vi "ke37xx Limit Test Results.vi"(0 "VISA Resource Name":refnum<visa-resource-name>, 7 "Clear (False)":bool, 11 "error in (no error)":errorcluster) -> (4 "VISA Resource Name Out":refnum<visa-resource-name>, 6 "Low Limit Failed":bool, 8 "High Limit Failed":bool, 15 "error out":errorcluster)   [LabVIEW 2009, in "Keithley 3700 Series.lvlib"]
doc: "This VI allows you to clear or to query the limit test results."
uses:
  <instrlib>/Keithley 3706/Keithley 3700 Series.lvlib
panel:
  in  "Limit Line (1)":u8=1 min=1 max=2
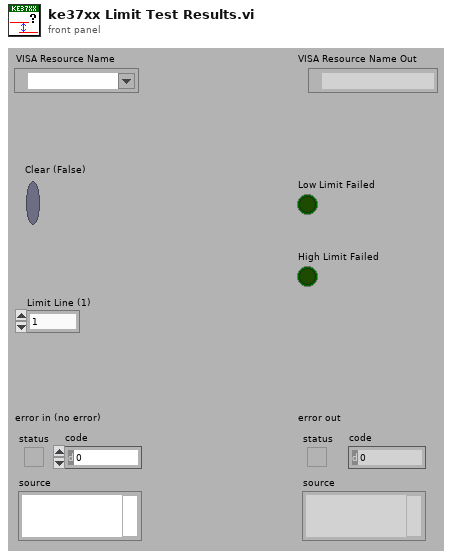
[diagram p1: front panel]
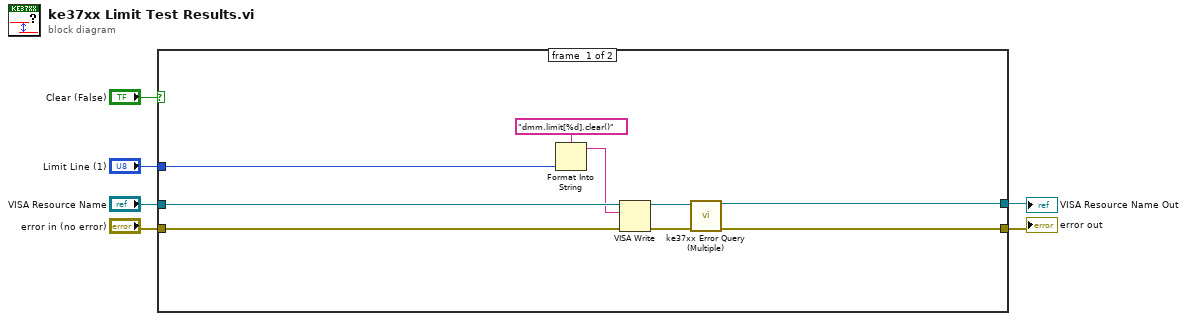
[diagram p0: block diagram]
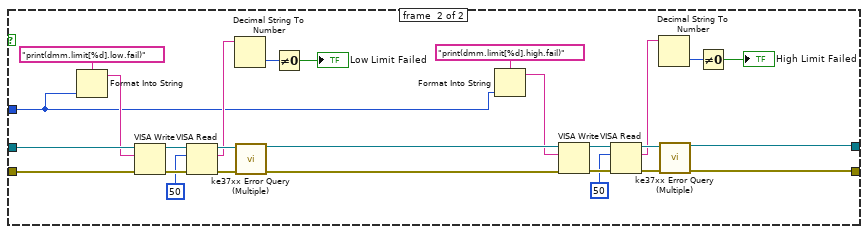
[diagram p2: hidden frame]
diagram:
  n1 = case shown="False" "Clear (False)" {
    tunnel: [w15 w18] -> w6
    tunnel: [w14 w16] -> w5
    tunnel: "VISA Resource Name" -> [w13 w39]
    tunnel: "error in (no error)" -> [w12 w38]
    tunnel: "Limit Line (1)" -> [w7 w20]
    frame #0 {
      n2 = Format Into String(format string="dmm.limit[%d].clear()", w7) -> (resulting string=w8:string)  [unwired: 2 in, 1 out]
      n3 = VISA Write(VISA resource name=w13, write buffer=w8, error in (no error)=w12) -> (VISA resource name out=w11:refnum<visa-resource-name>, error out=w10:errorcluster)  [unwired: 1 out]
      n4 = call <instrlib>:"ke37xx Error Query (Multiple).vi"("VISA resource name"=w11, "error in (no error)"=w10) -> ("VISA resource name out"=w15:refnum<visa-resource-name>, "error out"=w14:errorcluster)  [unwired: 12 out]
    }
    frame #1 {
      n5 = Format Into String(format string="print(dmm.limit[%d].low.fail)", w20) -> (resulting string=w36:string)  [unwired: 2 in, 1 out]
      n6 = VISA Write(VISA resource name=w39, write buffer=w36, error in (no error)=w38) -> (VISA resource name out=w35:refnum<visa-resource-name>, error out=w33:errorcluster)  [unwired: 1 out]
      n7 = VISA Read(VISA resource name=w35, byte count=u32 50, error in (no error)=w33) -> (VISA resource name out=w34:refnum<visa-resource-name>, read buffer=w30:string, error out=w32:errorcluster)  [unwired: 1 out]
      n8 = Decimal String To Number(string=w30) -> (number=w29:i32)  [unwired: 3 out]
      n9 = call <instrlib>:"ke37xx Error Query (Multiple).vi"("VISA resource name"=w34, "error in (no error)"=w32) -> ("VISA resource name out"=w42:refnum<visa-resource-name>, "error out"=w17:errorcluster)  [unwired: 12 out]
      n10 = Not Equal To 0?(x=w29) -> (x != 0?=→"Low Limit Failed":bool)
      n11 = Format Into String(format string="print(dmm.limit[%d].high.fail)", w20) -> (resulting string=w22:string)  [unwired: 2 in, 1 out]
      n12 = VISA Write(VISA resource name=w42, write buffer=w22, error in (no error)=w17) -> (VISA resource name out=w23:refnum<visa-resource-name>, error out=w40:errorcluster)  [unwired: 1 out]
      n13 = VISA Read(VISA resource name=w23, byte count=u32 50, error in (no error)=w40) -> (VISA resource name out=w41:refnum<visa-resource-name>, read buffer=w26:string, error out=w24:errorcluster)  [unwired: 1 out]
      n14 = Decimal String To Number(string=w26) -> (number=w27:i32)  [unwired: 3 out]
      n15 = call <instrlib>:"ke37xx Error Query (Multiple).vi"("VISA resource name"=w41, "error in (no error)"=w24) -> ("VISA resource name out"=w18:refnum<visa-resource-name>, "error out"=w16:errorcluster)  [unwired: 12 out]
      n16 = Not Equal To 0?(x=w27) -> (x != 0?=→"High Limit Failed":bool)
    }
  }
  "VISA Resource Name Out" <- w6
  "error out" <- w5
